vi "2Dto1DArray.vi"(2 "error in (no error)":errorcluster, 3 "Array In":dbl[][](array[numeric])) -> (0 "error out":errorcluster, 1 "Array Out":dbl[](array[numeric]))   [LabVIEW 2013, in "alpD41.lvlib"]
uses:
  alpD41.lvlib
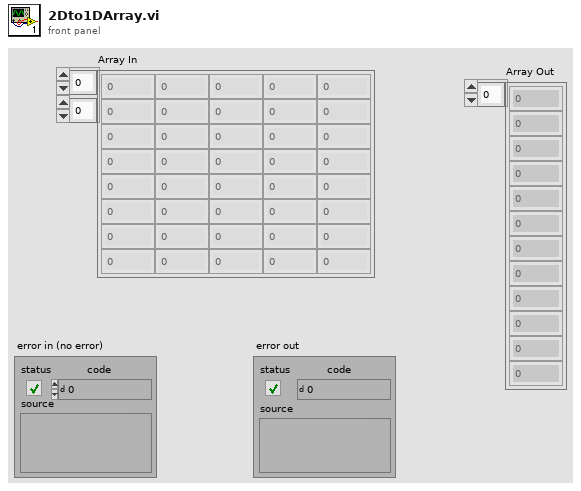
[diagram p1: front panel]
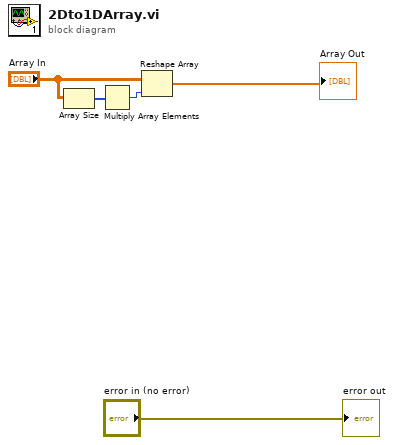
[diagram p0: block diagram]
diagram:
  n1 = Array Size(array="Array In") -> (size(s)=w5:i32[])
  n2 = Multiply Array Elements(1:w5) -> (0:w4:i32)
  n3 = Reshape Array("Array In", w4) -> (→"Array Out":dbl[])
  "error out" <- "error in (no error)"
